vi "RoughTerrain_Drive_Back.vi"(0 "Auto_Selection":T2=enum."Ramparts", 1 "Encoder":dbl=239.29603649999999, 2 "Yaw":dbl=105.81992569508552, 3 "Dist_Foward":dbl=303.0670068027601, 4 "Auto_Enable":bool) -> (5 "Motor Speed":dbl, 6 "Rest_Encoder":bool, 7 "Rest_Gyro":bool, 8 "Rough Terrain On":bool, 9 "Intake Arm Lowered":bool)   [LabVIEW 2015]
uses:
  Auto_Selection.ctl
  AutoEnum.ctl
panel:
  out "Shooter_Speed":dbl
  out "Shoot":bool
  out "Stage":bool
  in  "Moat_Speed 2":dbl=-1.0 format="%#_13g"
  in  "Pamparts_Speed 2":dbl=-0.75 format="%#_13g"
  in  "Rock_Wall_Speed 2":dbl=-1.0 format="%#_13g"
  in  "Rough_Speed 2":dbl=-0.75 format="%#_13g"
  in  "Numeric 2":i32=10000
  in  "Min_Dist_Drive 2":dbl=50.0
  in  "DB_Pitch 2":dbl=4.0
  in  "DB_Pitch":dbl=4.0
  in  "Min_Pitch":dbl=3.0
  in  "Min_Dist_Drive":dbl=50.0
  in  "Return_Enable":bool
  in  "Pitch":dbl=105.81992569508552
  in  "Numeric":i32=10000
  in  "Distaince_DB":dbl=1.0
  out "error":errorcluster={"status"=TRUE, "code"=0, "source"="DID NOT DRIVE THE DISTANCE : ROUGH TERRAIN"}
  out "Enum":T1
  out "x = y?":bool
  in  "Distance Goal":dbl=180.0
  in  "Pamparts_Speed":dbl=-0.75 format="%#_13g"
  in  "Rock_Wall_Speed":dbl=-1.0 format="%#_13g"
  in  "Rough_Speed":dbl=-0.75 format="%#_13g"
  in  "Moat_Speed":dbl=-1.0 format="%#_13g"
  in  "Clear Error":bool
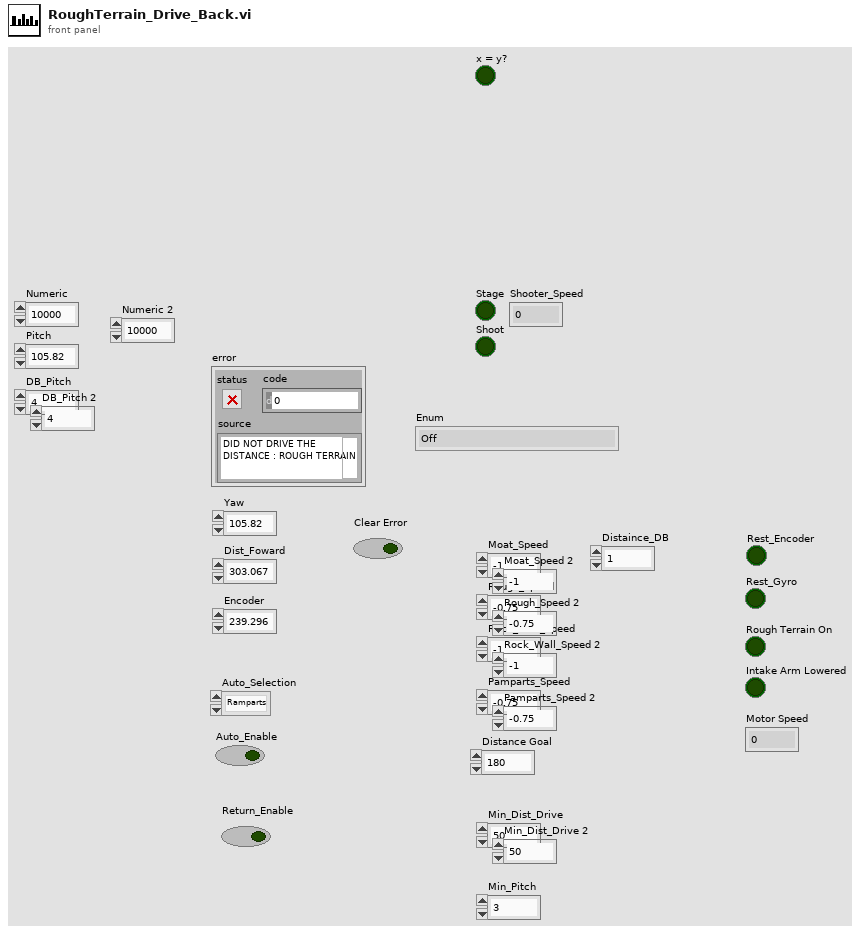
[diagram p1: front panel]
types:
  T1 = typedef "AutoEnum.ctl" = enum16{"Off", "ResetVar", "ResetOff", "BeforeTeeter", "LowerArm", "DriveForward", "Stop", "Stop One", "Drive Back", "Drive Forward Two"}
  T2 = typedef "Auto_Selection.ctl" = enum16{"Low Bar", "Rough Terrain", "Rock Wall", "Ramparts", "Moat", "Cheval de Frise", "Portcullis", "None", "One  Ball"}
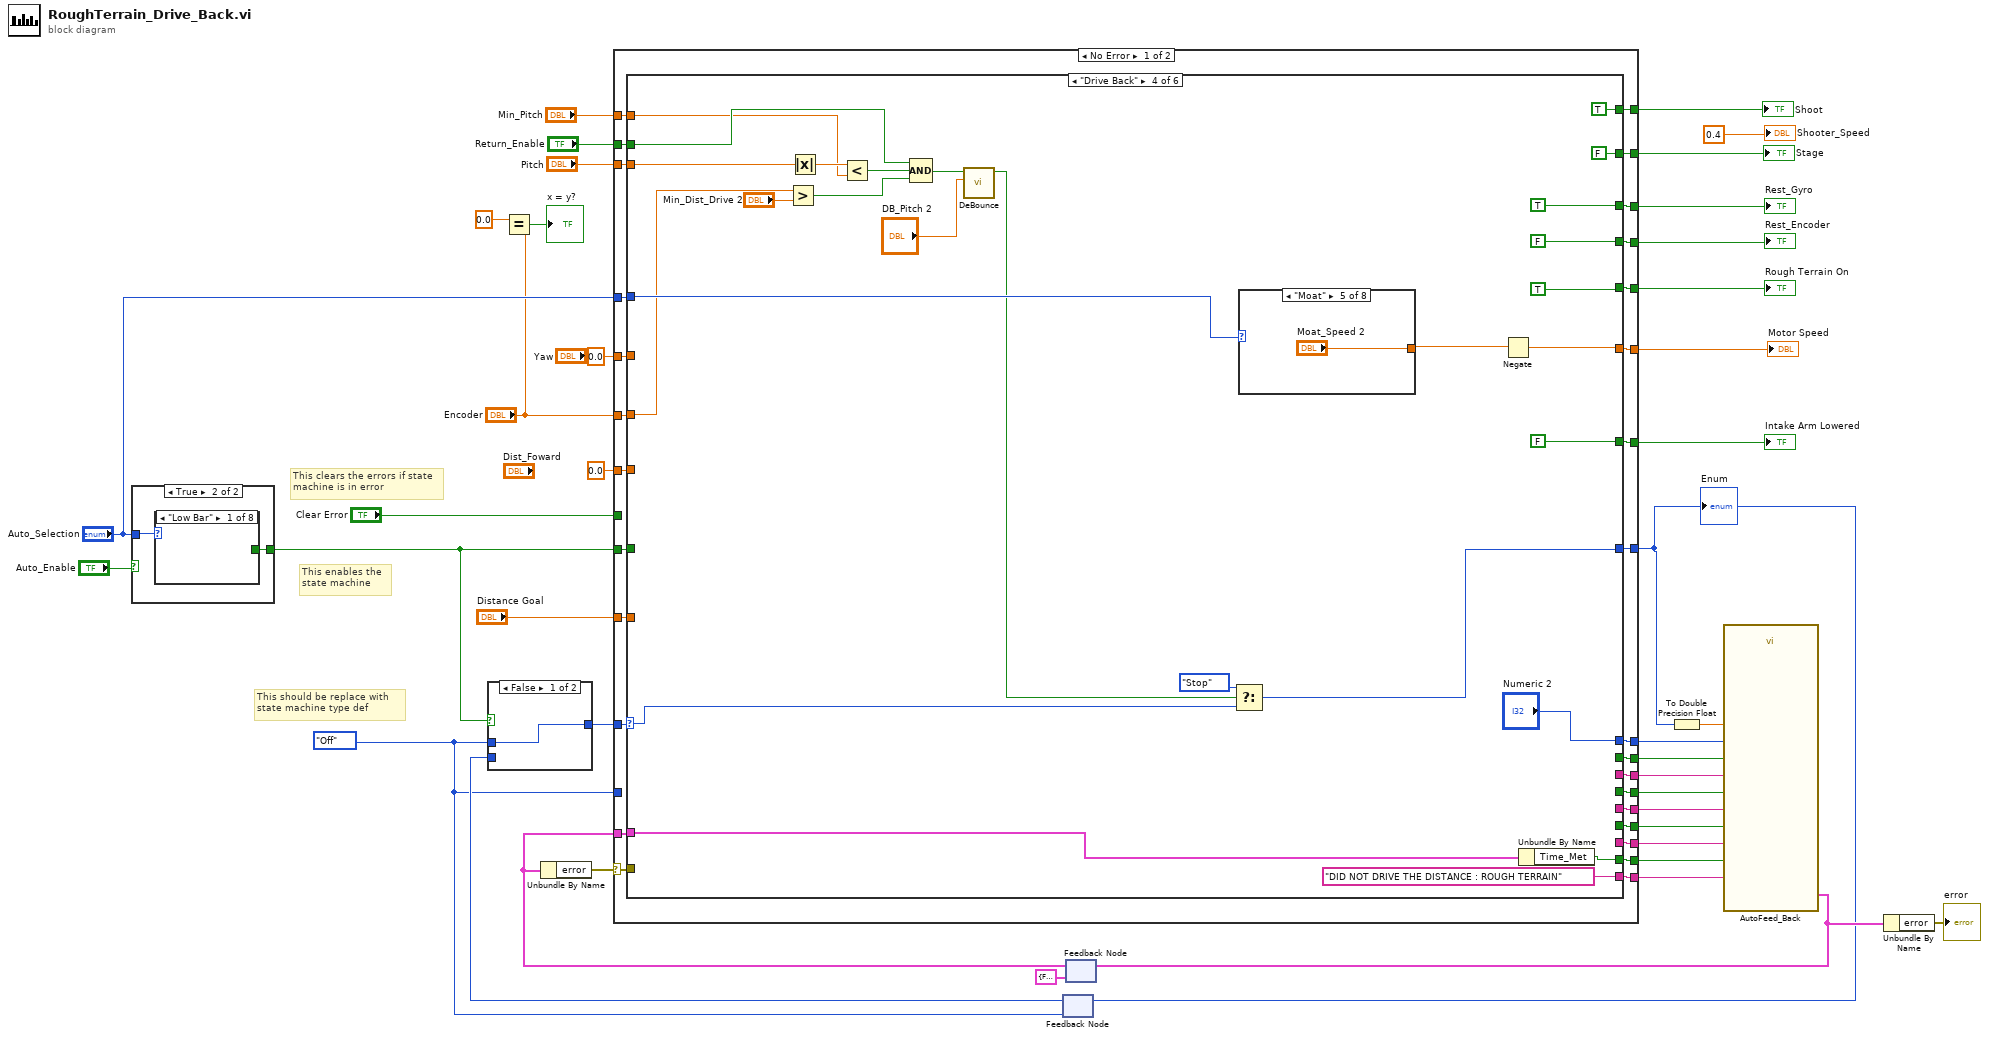
[diagram p0: block diagram]
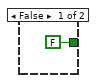
[diagram p2: hidden frame]
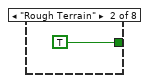
[diagram p3: hidden frame]
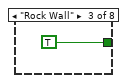
[diagram p4: hidden frame]
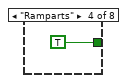
[diagram p5: hidden frame]
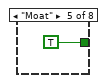
[diagram p6: hidden frame]
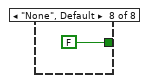
[diagram p9: hidden frame]
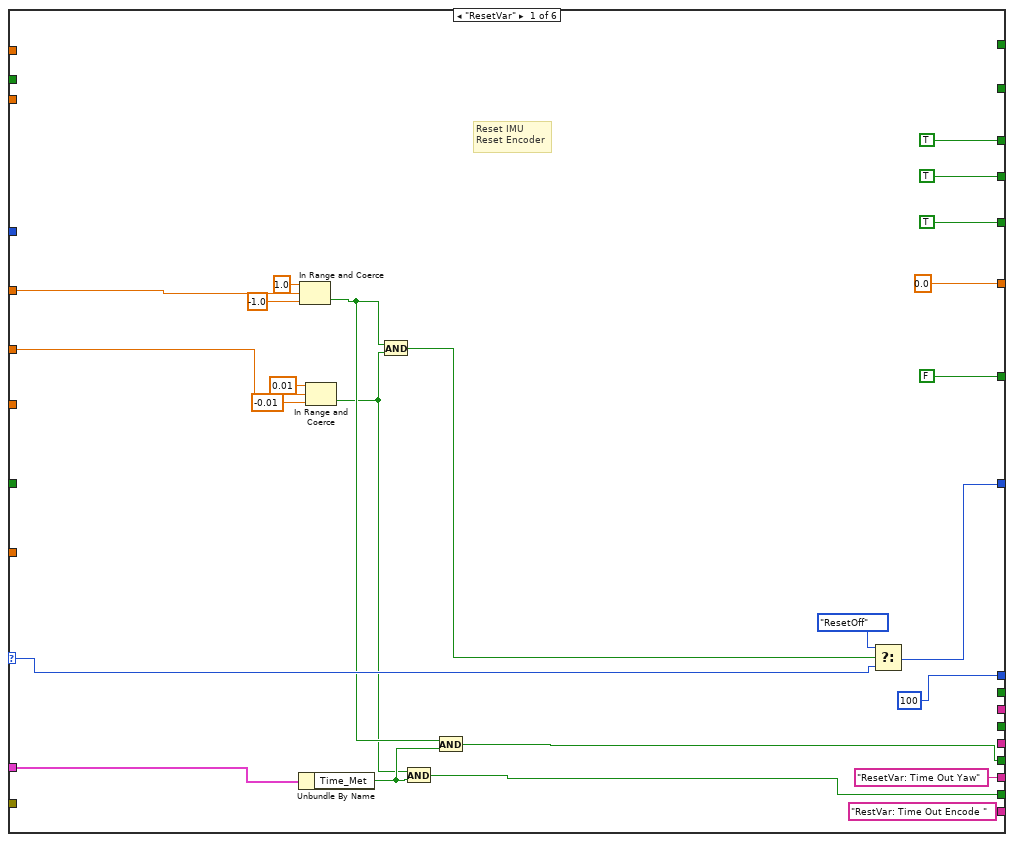
[diagram p11: hidden frame]
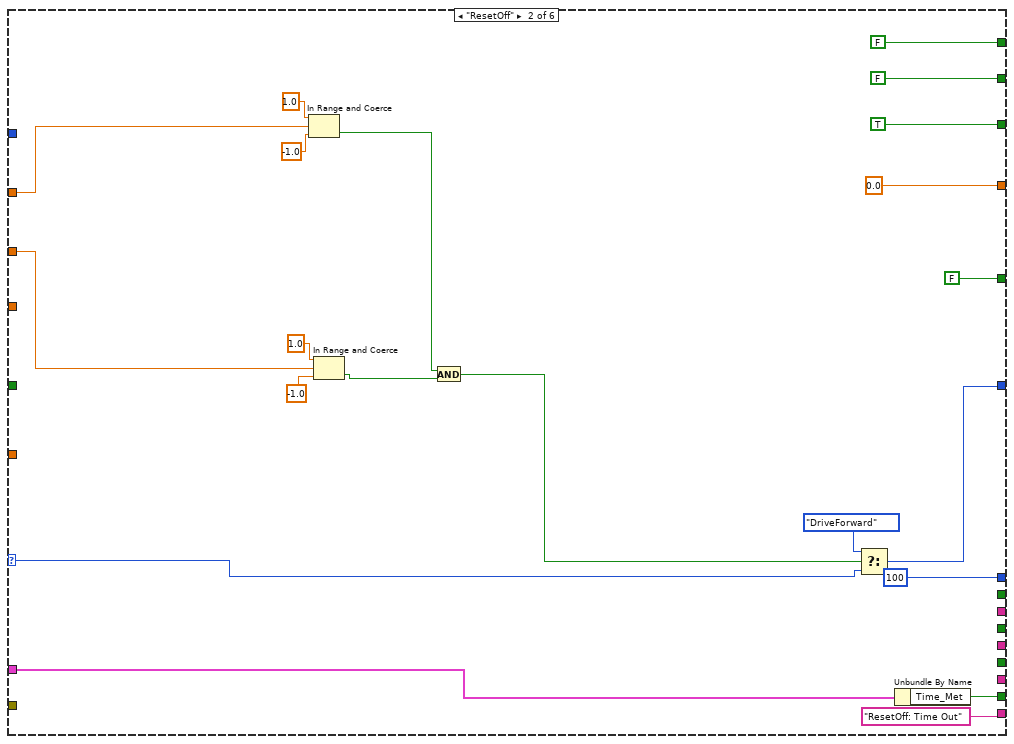
[diagram p12: hidden frame]
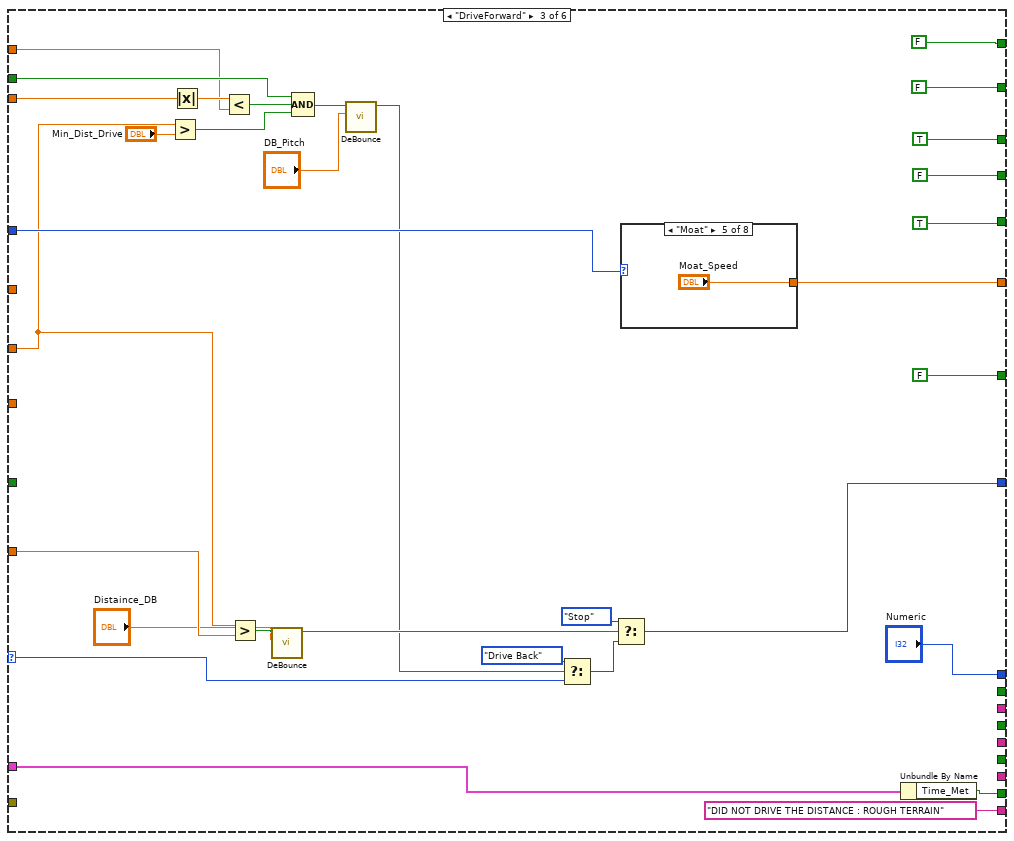
[diagram p13: hidden frame]
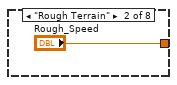
[diagram p15: hidden frame]
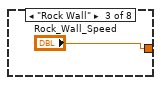
[diagram p16: hidden frame]
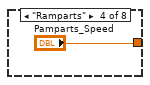
[diagram p17: hidden frame]
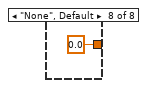
[diagram p20: hidden frame]
diagram:
  w30 = AutoEnum."Off"
  # "This clears the errors if state \nmachine is in error"
  # "This enables the \nstate machine"
  # "This should be replace with \nstate machine type def"
  n1 = case shown="True" "Auto_Enable" {
    tunnel: "Auto_Selection" -> [_ w43]
    tunnel: [FALSE w42] -> w26
    frame False {
    }
    frame True {
      n2 = case shown="\"Low Bar\"" w43 {
        tunnel: [_ TRUE TRUE TRUE TRUE _ _ FALSE] -> w42
        frame "Low Bar" {
        }
        frame "Rough Terrain" {
        }
        frame "Rock Wall" {
        }
        frame "Ramparts" {
        }
        frame "Moat" {
        }
        frame "Cheval de Frise" {
        }
        frame "Portcullis" {
        }
        frame "None", Default {
        }
      }
    }
  }
  n3 = Equal?(x=0.0, y="Encoder") -> (x = y?=→"x = y?":bool)
  n4 = feedback #1(w30) -> (w32:T1)
  n5 = case shown="False" w26 {
    tunnel: w30 -> [w49 _]
    tunnel: [w49 w50] -> w33
    tunnel: w32 -> [_ w50]
    frame False {
    }
    frame True {
    }
  }
  n6 = feedback #2(cluster{"Time_Met":bool, "error ":errorcluster} {"Time_Met"=FALSE, "error "={"status"=FALSE, "code"=0, "source"=""}} ("Feedback_State")) -> (w34:cluster{"Time_Met":bool, "error ":errorcluster})
  n7 = Unbundle By Name(w34) -> ("error"=w36:errorcluster)
  n8 = case shown="No Error" w36 {
    selector: w36 -> [w74 w238]
    tunnel: [w79 FALSE] -> w40
    tunnel: [w78 FALSE] -> w39
    tunnel: [w77 w235] -> w10
    tunnel: [w76 0] -> w38
    tunnel: "Clear Error" -> [_ w237]
    tunnel: w34 -> [w75 _]
    tunnel: w26 -> [w73 _]
    tunnel: w33 -> [w72 _]
    tunnel: w30 -> [_ w235]
    tunnel: [w71 0.0] -> w29
    tunnel: [w70 FALSE] -> w28
    tunnel: [w69 FALSE] -> w27
    tunnel: 0.0 ("Yaw") -> [w68 _]
    tunnel: "Encoder" -> [w67 _]
    tunnel: 0.0 ("Dist_Foward") -> [w66 _]
    tunnel: "Auto_Selection" -> [w65 _]
    tunnel: [w64 w230] -> w23
    tunnel: [w63 FALSE] -> w22
    tunnel: [w62 FALSE] -> w21
    tunnel: [w61 FALSE] -> w20
    tunnel: [w60 w229] -> w19
    tunnel: [w59 ""] -> w18
    tunnel: [w58 ""] -> w17
    tunnel: [w57 ""] -> w16
    tunnel: "Distance Goal" -> [w56 _]
    tunnel: "Pitch" -> [w55 _]
    tunnel: "Return_Enable" -> [w54 _]
    tunnel: "Min_Pitch" -> [w53 _]
    tunnel: [w52 FALSE] -> w3
    tunnel: [w51 FALSE] -> w2
    frame No Error {
      n9 = case shown="\"Drive Back\"" w72 {
        selector: w72 -> [w95 w118 w129 w162 _ w216]
        tunnel: [TRUE FALSE TRUE TRUE FALSE FALSE] -> w79
        tunnel: [TRUE FALSE FALSE FALSE FALSE FALSE] -> w78
        tunnel: [100 100 "Numeric" "Numeric 2" 2000 0] -> w76
        tunnel: [w94 w117 w143 w179 AutoEnum."Stop" w215] -> w77
        tunnel: w75 -> [w97 w108 w144 w180 _ _]
        tunnel: w74 -> [_ _ _ _ _ _]
        tunnel: w73 -> [_ _ _ _ _ w217]
        tunnel: [0.0 0.0 w149 w166 0.0 0.0] -> w71
        tunnel: [TRUE TRUE TRUE TRUE FALSE FALSE] -> w70
        tunnel: [FALSE FALSE FALSE FALSE FALSE FALSE] -> w69
        tunnel: w68 -> [w83 w110 _ _ _ _]
        tunnel: w67 -> [w82 w109 w140 w177 _ _]
        tunnel: w66 -> [_ _ _ _ _ _]
        tunnel: w65 -> [_ _ w150 w182 _ _]
        tunnel: [_ _ _ _ _ FALSE] -> w64
        tunnel: [_ _ _ _ _ FALSE] -> w63
        tunnel: [w81 _ _ _ _ FALSE] -> w62
        tunnel: [w80 w105 w141 w178 _ FALSE] -> w61
        tunnel: [_ _ _ _ _ ""] -> w60
        tunnel: [_ _ _ _ _ ""] -> w59
        tunnel: ["ResetVar: Time Out Yaw" _ _ _ _ ""] -> w58
        tunnel: ["RestVar: Time Out Encode " ("source") "ResetOff: Time Out" ("source") "DID NOT DRIVE THE DISTANCE : ROUGH TERRAIN" ("source") "DID NOT DRIVE THE DISTANCE : ROUGH TERRAIN" ("source") _ ""] -> w57
        tunnel: w56 -> [_ _ w147 _ _ _]
        tunnel: w55 -> [_ _ w138 w175 _ _]
        tunnel: w54 -> [_ _ w133 w170 _ _]
        tunnel: w53 -> [_ _ w127 w168 _ _]
        tunnel: [_ _ FALSE FALSE _ FALSE] -> w52
        tunnel: [_ _ FALSE TRUE _ FALSE] -> w51
        frame "ResetVar" {
          # "Reset IMU\nReset Encoder"
          n10 = Unbundle By Name(w97) -> ("Time_Met"=w89:bool)
          n11 = In Range and Coerce(upper limit=1.0, x=w83, lower limit=-1.0) -> (In Range?=w88:bool)  [unwired: 1 out]
          n12 = In Range and Coerce(upper limit=0.01, x=w82, lower limit=-0.01) -> (In Range?=w84:bool)  [unwired: 1 out]
          n13 = And(x=w88, y=w84) -> (x .and. y?=w93:bool)
          n14 = And(x=w84, y=w89) -> (x .and. y?=w80:bool)
          n15 = And(x=w88, y=w89) -> (x .and. y?=w81:bool)
          n16 = Select(t=AutoEnum."ResetOff", s=w93, f=w95) -> (s? t:f=w94:T1)
        }
        frame "ResetOff" {
          n17 = In Range and Coerce(upper limit=1.0, x=w110, lower limit=-1.0) -> (In Range?=w113:bool)  [unwired: 1 out]
          n18 = In Range and Coerce(upper limit=1.0, x=w109, lower limit=-1.0) -> (In Range?=w111:bool)  [unwired: 1 out]
          n19 = And(x=w113, y=w111) -> (x .and. y?=w107:bool)
          n20 = Select(t=AutoEnum."DriveForward", s=w107, f=w118) -> (s? t:f=w117:T1)
          n21 = Unbundle By Name(w108) -> ("Time_Met"=w105:bool)
        }
        frame "DriveForward" {
          n22 = Greater?(x=w140, y="Min_Dist_Drive") -> (0:w135:bool)
          n23 = Absolute Value(x=w138) -> (abs(x)=w137:dbl)
          n24 = Less?(x=w137, y=w127) -> (x < y?=w136:bool)
          n25 = Greater?(x=w140, y=w147) -> (0:w146:bool)
          n26 = call "DeBounce.vi"("DB_Count"="Distaince_DB", "Value"=w146) -> ("BD_Value"=w142:bool)  [unwired: 9 in]
          n27 = Compound Arithmetic op=AND(w133, w136, w135) -> (w132:bool)
          n28 = call "DeBounce.vi"("DB_Count"="DB_Pitch", "Value"=w132) -> ("BD_Value"=w130:bool)  [unwired: 9 in]
          n29 = Select(t=AutoEnum."Drive Back", s=w130, f=w129) -> (s? t:f=w131:T1)
          n30 = Select(t=AutoEnum."Stop", s=w142, f=w131) -> (s? t:f=w143:T1)
          n31 = case shown="\"Moat\"" w150 {
            tunnel: [_ "Rough_Speed" "Rock_Wall_Speed" "Pamparts_Speed" "Moat_Speed" _ _ 0.0 ("Moat_Speed")] -> w149
            frame "Low Bar" {
            }
            frame "Rough Terrain" {
            }
            frame "Rock Wall" {
            }
            frame "Ramparts" {
            }
            frame "Moat" {
            }
            frame "Cheval de Frise" {
            }
            frame "Portcullis" {
            }
            frame "None", Default {
            }
          }
          n32 = Unbundle By Name(w144) -> ("Time_Met"=w141:bool)
        }
        frame "Drive Back" {
          n33 = Greater?(x=w177, y="Min_Dist_Drive 2") -> (0:w172:bool)
          n34 = Absolute Value(x=w175) -> (abs(x)=w174:dbl)
          n35 = Less?(x=w174, y=w168) -> (x < y?=w173:bool)
          n36 = Compound Arithmetic op=AND(w170, w173, w172) -> (w169:bool)
          n37 = call "DeBounce.vi"("DB_Count"="DB_Pitch 2", "Value"=w169) -> ("BD_Value"=w163:bool)  [unwired: 9 in]
          n38 = Select(t=AutoEnum."Stop", s=w163, f=w162) -> (s? t:f=w179:T1)
          n39 = case shown="\"Moat\"" w182 {
            tunnel: [_ "Rough_Speed 2" "Rock_Wall_Speed 2" "Pamparts_Speed 2" "Moat_Speed 2" _ _ 0.0 ("Moat_Speed")] -> w167
            frame "Low Bar" {
            }
            frame "Rough Terrain" {
            }
            frame "Rock Wall" {
            }
            frame "Ramparts" {
            }
            frame "Moat" {
            }
            frame "Cheval de Frise" {
            }
            frame "Portcullis" {
            }
            frame "None", Default {
            }
          }
          n40 = Negate(x=w167) -> (-x=w166:dbl)
          n41 = Unbundle By Name(w180) -> ("Time_Met"=w178:bool)
        }
        frame "Stop" {
        }
        frame "Off", Default {
          # "Nothing : Everything Off"
          n42 = Select(t=AutoEnum."ResetVar", s=w217, f=w216) -> (s? t:f=w215:T1)
        }
      }
    }
    frame Error {
      n43 = Select(t=errorcluster {"status"=FALSE, "code"=0, "source"=""}, s=w237, f=w238) -> (s? t:f=w231:errorcluster)
      n44 = Unbundle By Name(w231) -> ("status"=w230:bool, "source"=w229:string)
    }
  }
  "Rest_Gyro" <- w40
  "Rest_Encoder" <- w39
  "Motor Speed" <- w29
  "Rough Terrain On" <- w28
  "Intake Arm Lowered" <- w27
  "Enum" <- w10
  "Stage" <- w3
  "Shoot" <- w2
  n45 = feedback-in #1(w10) -> ()
  n46 = To Double Precision Float(number=w10) -> (double precision float=w31:dbl)
  n47 = call "AutoFeed_Back.vi"("Code 4"=w16, "Error_4_En"=w20, "Code 3"=w17, "Code 2"=w18, "Error_3_En"=w21, "Error_2_En"=w22, "Code 1"=w19, "Error_1_En"=w23, "Time (ms)"=w38, "State"=w31) -> ("Feedback_State"=w12:cluster{"Time_Met":bool, "error ":errorcluster})  [unwired: 1 in]
  n48 = feedback-in #2(w12) -> ()
  n49 = Unbundle By Name(w12) -> ("error"=→"error":errorcluster)
  "Shooter_Speed" <- 0.4
